vi "Send Message to Queue.vi"() -> ()   [LabVIEW 2015]
doc: "Demonstrates how to send a message to an existing Amazon SQS queue."
uses:
  Core/HTTP Request/Region.ctl
  Core/HTTP Request/AWS Credentials.ctl
  Queue/Queue.lvclass
  Core/HTTP Request/HTTP Request.lvclass
panel:
  in  "Region":T1
  in  "Secret Key":string
  in  "Access Key":string
  in  "Queue Name":string
  in  "Message Body":string
  # "Overview: Demonstrates how to send a message to an existing Amazon SQS queue.\nRequirements: LabVIEW AWS Toolkit and a registered Amazon AWS account\nInstructions:\n1. Specify the Access Key and Secret Key for your AWS account. You can create an account at http://aws.amazon.com.\n2. Specify a Region and Queue Name for the queue to which you want to send a message.\n3. Specify a Message Body to send to the queue.\n4. Run the VI. Verify in the Amazon SQS console that the specified queue has an available message."
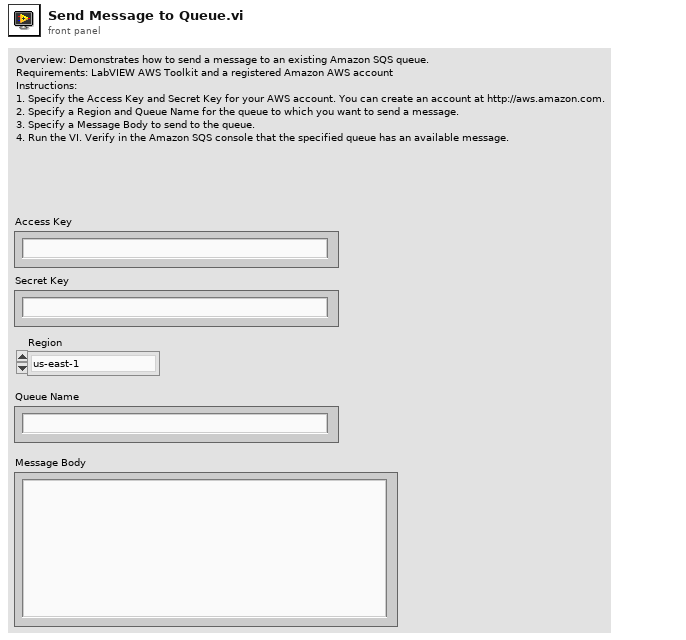
[diagram p1: front panel]
types:
  T1 = typedef "NI_AWS_Core.lvlib/HTTP Request.lvclass/Region.ctl" = enum16{"us-east-1", "us-east-2", "us-west-1", "us-west-2", "ap-northeast-1", "ap-northeast-2", "ap-southeast-1", "ap-southeast-2", "ca-central-1", "eu-central-1", "eu-west-1", "eu-west-2", "sa-east-1"}
  T2 = typedef "NI_AWS_Core.lvlib/HTTP Request.lvclass/AWS Credentials.ctl" = cluster{"Access Key":string, "Secret Key":string}
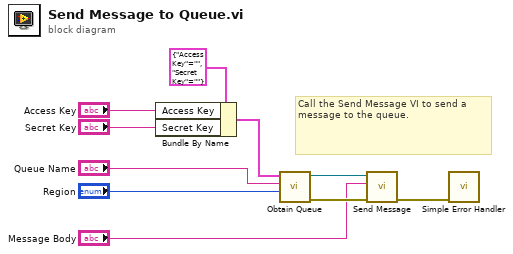
[diagram p0: block diagram]
diagram:
  # "Call the Send Message VI to send a message to the queue."
  n1 = Bundle By Name(cluster=T2 {"Access Key"="", "Secret Key"=""} ("AWS Credentials"), "Access Key"="Access Key", "Secret Key"="Secret Key") -> (w4:T2)
  n2 = call "Obtain Queue.vi"("Region"="Region", "Name"="Queue Name", "AWS Credentials"=w4) -> ("error out"=w9:errorcluster, "SQS"=w10:refnum<class "Queue.lvclass">)  [unwired: 7 in]
  n3 = call "Send Message.vi"("error in (no error)"=w9, "Message Body"="Message Body", "SQS in"=w10) -> ("error out"=w8:errorcluster)  [unwired: 4 in, 4 out]
  n4 = call <vilib>:"Simple Error Handler.vi"("error in (no error)"=w8) -> ()  [unwired: 4 in, 5 out]
